vi "Dashboard Main.vi"() -> ()   [LabVIEW 2013]
uses:
  <vilib>/event_ctls.llb/eventvkey.ctl
  <vilib>/Rock Robotics/WPI/Dashboard/WPI_DashboardLogging Global.vi
  <vilib>/Utility/config.llb/Write Key (String).vi
  <vilib>/Utility/config.llb/Write Key (I32).vi
  <vilib>/Utility/config.llb/NI_LVConfig.lvlib
panel:
  out "Image Message":string="Timeout in Camera Communications"
  in  "Rec Mode":enum32{"Stop", "Record", "Playback"}(radio)
  in  "Dashboard Tab":T1(tab)
  in  "Camera Settings":T2={"Frame Rate"=30, "Compression"=30, "Size"=1} {"Frame Rate" scale=1.0..30.0; "Size" items=["640x480", "320x240", "160x120"]}
  out "MotorSliders R":cluster{"MotorSlide1":dbl, "MotorSlide2":dbl} {"MotorSlide2" scale=-1.0..1.0 scale format="%#_2e"; "MotorSlide1" scale=-1.0..1.0 scale format="%#_2e"}
  out "MotorChart R":cluster{"Numeric":dbl, "Numeric":dbl}(graph)
  out "MotorSliders L":T3 {"MotorSlide4 2" scale=0.0..14.0 scale format="%#_2e"; "MotorSlide2" scale=-1.0..1.0 scale format="%#_2e"; "MotorSlide1" scale=-1.0..1.0 scale format="%#_2e"}
  out "MotorChart L":T4(graph)
  out "JS1 Z":dbl(slide) scale=-1.0..1.0 scale format="%#_2e"
  out "Joystick 1":cluster{"X":dbl, "Y":dbl}[](graph)
  out "JS Buttons 1":T5
  out "JS2 Z":dbl(slide) scale=-1.0..1.0 scale format="%#_2e"
  out "Joystick 2":cluster{"X":dbl, "Y":dbl}[](graph)
  out "JS Buttons 2":T5
  out "Mode":T6(ring)=enum."Auto Disabled"
  out "Camera IP":string
  in  "DB Camera Config":bool
  out "fps":dbl format="%#.1g"
  out "Mbps":dbl format="%#.1g"
  out "Mbps 2":bool
  out "LED 1":bool
  in  "Light Ring On":bool
  in  "Drawback Pistons Activated":bool
  out "Buttons Of Same Pistons In Same State":bool
  in  "Compressor On/Off":bool
  in  "Grabber Pistons Extended":bool
  out "Are Grabber Pistons Extended":bool
  in  "Camera Pitch Control":dbl
  in  "Camera Rotation Control":dbl
  out "Is The Firing Pin Piston Extended":bool
  out "Are Drawback Pistons Extended":bool
  in  "Firing Pin Piston Extended":bool
  in  "Drawback Piston Extended":bool
  in  "Manual Mechanism Override":bool
  in  "Current Grabber Status":enum16{""}(ring)
  in  "Current Shooter Status":enum16{""}(ring)
  in  "Checkbox 2":bool
  in  "Checkbox 1":bool
  in  "Test Slider":dbl(slide) scale=0.0..100.0 scale format="%#_3g"
  in  "On/Off":bool caption="Solenoid"
  in  "Test Name":u16(ring) items=["Select the test to run...", "Example Test", "-------------------------------", "List of tests is built in robot code.", "Replace with your own automated tests."]
  in  "Test Tree":string(tree)
  in  "Motor":cluster{"Value":dbl, "Enable":bool} {"Value" scale=-1.0..1.0 scale format="%#_3g"}
  out "Progress":T7 {"Test Progress" scale=0.0..100.0}
  in  "Rev/Fwd":cluster{"Forward":bool, "Reverse":bool}
  in  "Test Ring":u16(ring) items=["Auto", "Fixed indoor", "Fixed outdoor 1", "Fixed outdoor 2", "Fixed fluorescent 1", "Fixed fluorescent 2", "Hold current"]
  in  "Listbox":i32(listbox)
  out "Tree":string(tree)
  out "Camera Image":T8(plugin-control)
  in  "Enable":bool
  # "Left"
  # "Front"
  # "Right"
  # "Battery"
  # "Don5"
  # "This tab is a great place for autonomous settings and validation.\nCustomize by placing controls and indicators here and name to\nmatch Dashboard Variables on robot."
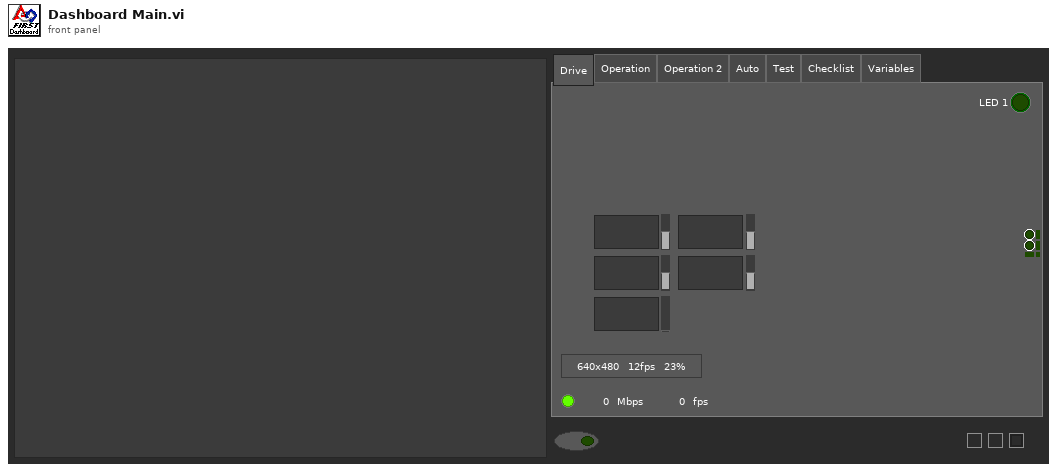
[diagram p1: front panel]
types:
  T1 = enum32{"Drive", "Operation", "Operation 2", "Auto", "Test", "Checklist", "Variables"}
  T2 = cluster{"Frame Rate":i32, "Compression":i32, "Size":u16}
  T3 = cluster{"MotorSlide1":dbl, "MotorSlide2":dbl, "MotorSlide4 2":dbl}
  T4 = cluster{"Numeric":dbl, "Numeric":dbl, "Battery":sgl}
  T5 = cluster{bool, bool, bool, bool, bool, bool, bool, bool, bool, bool, bool, bool}
  T6 = enum8{"Tele-Op Disabled", "Tele-Op Enabled", "Auto Disabled", "Auto Enabled", "Test Disabled", "Test Enabled", ""}
  T7 = cluster{"Test Progress":u8, "Test Progress Text":string}
  T8 = typedef "IMAQ Image.ctl" = refnum<image>
  T9 = enum32{"Drive", "Operation", "Auto", "Test", "Checklist", "Variables"}
  T10 = typedef "Image Type" = u32
  T11 = cluster{"Digital Inputs":bool[], "Digital Outputs":bool[]}
  T12 = cluster{"Competition mode":bool, "Robot Link":bool, "Autonomous":bool, "Enabled":bool, "E-Stop":bool, "Simulated":bool, "TestMode":bool, "Docked Window":bool}
  T13 = cluster{"Boolean Array[0]":bool, "Boolean Array[1]":bool, "Boolean Array[2]":bool, "Boolean Array[3]":bool, "Boolean Array[4]":bool, "Boolean Array[5]":bool, "Boolean Array[6]":bool, "Boolean Array[7]":bool, "Boolean Array[8]":bool, "Boolean Array[9]":bool, "Boolean Array[10]":bool, "Boolean Array[11]":bool}
  T14 = typedef "NI_LVConfig.lvlib/Config Data RefNum.ctl" = refnum<k1>
  T15 = typedef "eventvkey.ctl" = enum16{"ASCII", "Enter", "Return", "Shift", "Ctrl", "Alt", "Cmd", "Opt", "Caps", "NumLock", "Clear", "Break", "Up", "Down", "Left", "Right", "Insert", "Delete", "Home", "End", "PageUp", "PageDown", "Escape", "Help", "Pause", "ScrollLock", "F1", "F2", "F3", "F4", "F5", "F6", "F7", "F8", "F9", "F10", "F11", "F12", "F13", "F14", "F15", "F16", "F17", "F18", "F19", "F20", "F21", "F22", "F23", "F24", "Play", "VolumeUp", "VolumeDown", "Mute", "Two Byte Char"}
  T16 = cluster{"Image Size":bool, "Image Type":bool, "Pixel Value":bool, "ROI Information":bool, "Zoom Factor":bool}
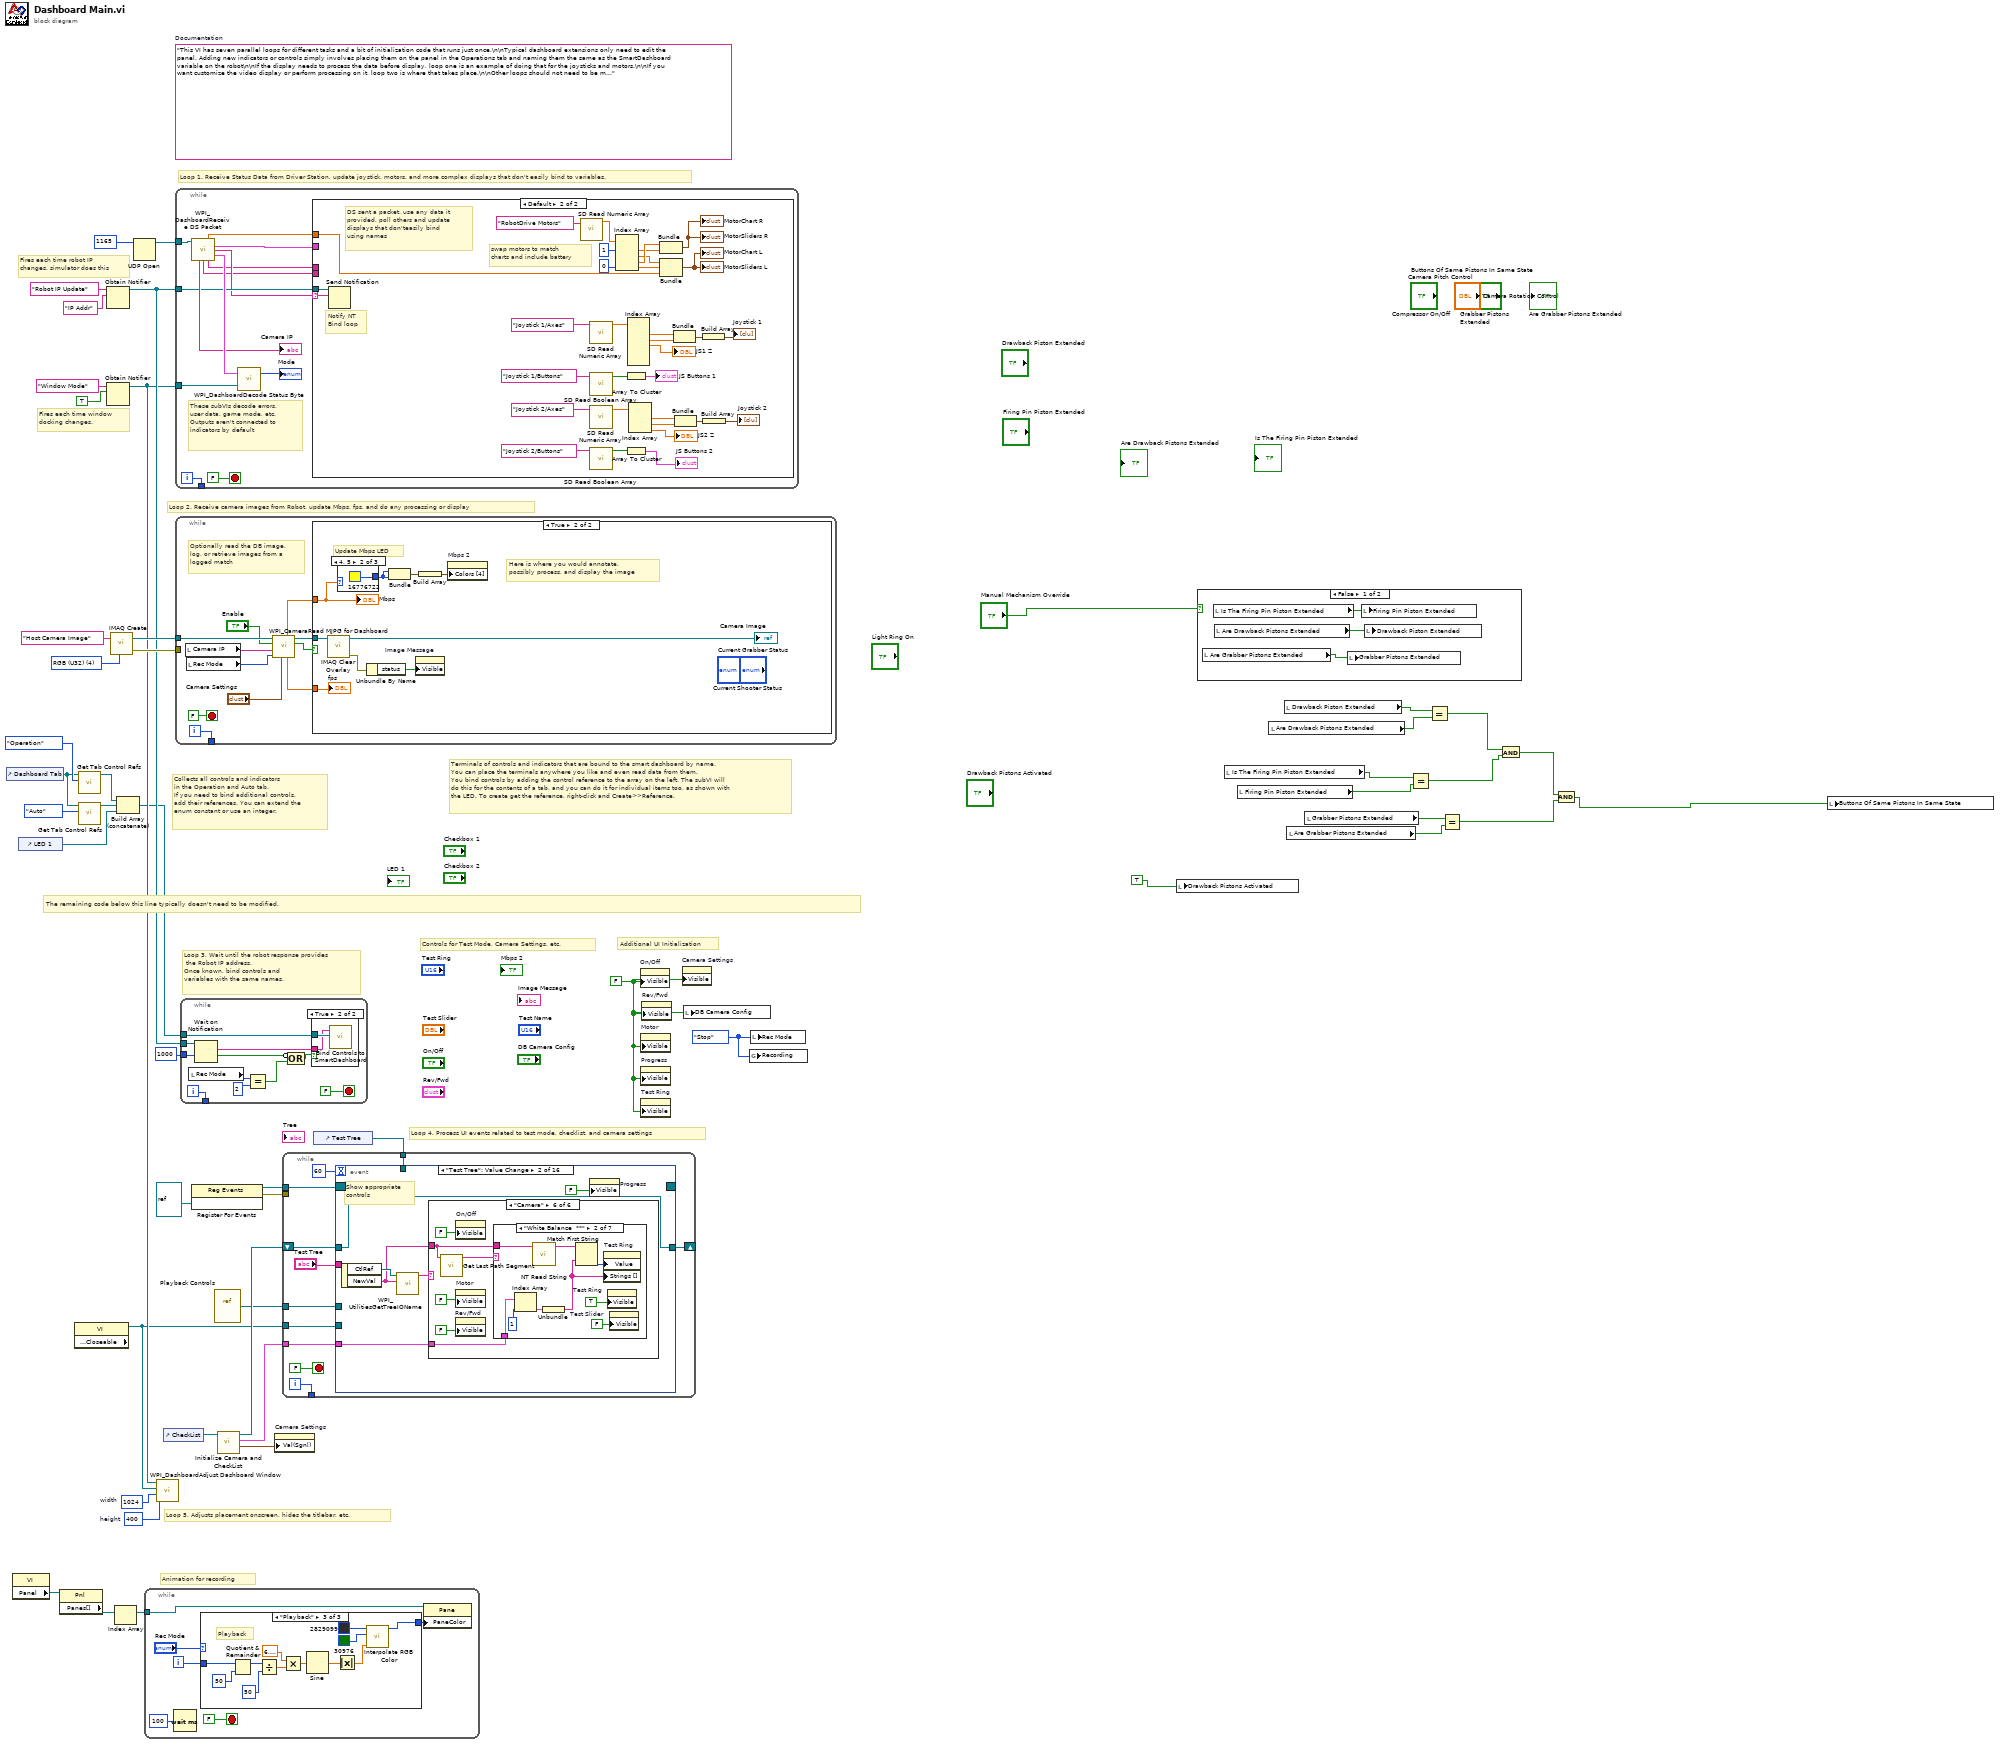
[diagram p0: block diagram]
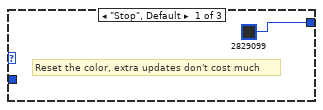
[diagram p3: hidden frame]
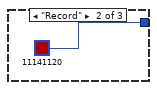
[diagram p4: hidden frame]
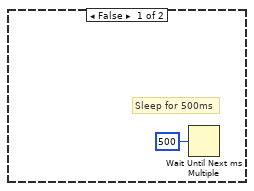
[diagram p6: hidden frame]
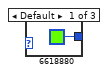
[diagram p7: hidden frame]
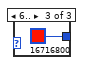
[diagram p8: hidden frame]
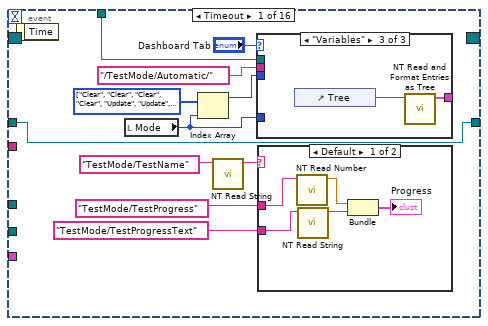
[diagram p9: hidden frame]
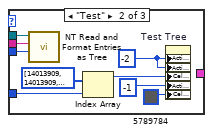
[diagram p11: hidden frame]
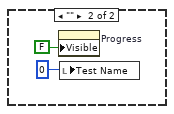
[diagram p12: hidden frame]
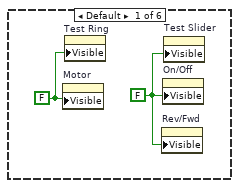
[diagram p13: hidden frame]
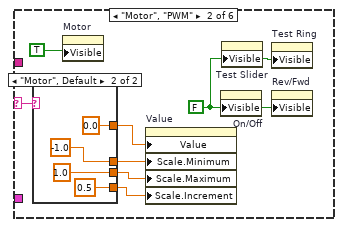
[diagram p14: hidden frame]
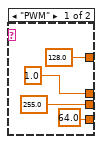
[diagram p15: hidden frame]
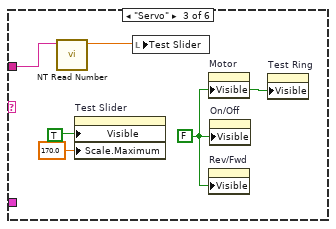
[diagram p16: hidden frame]
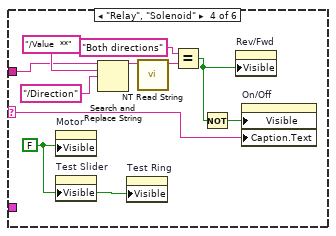
[diagram p17: hidden frame]
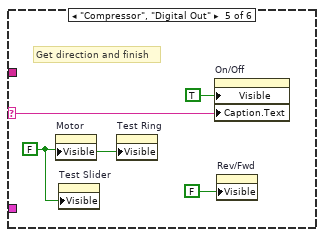
[diagram p18: hidden frame]
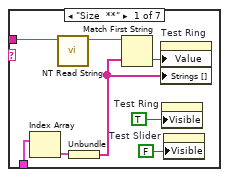
[diagram p19: hidden frame]
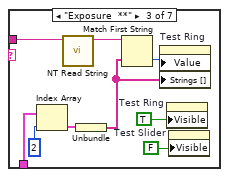
[diagram p20: hidden frame]
diagram:
  w21 = enum32{"Stop", "Record", "Playback"}."Stop" ("Rec Mode")
  w24 = 400  # height
  w25 = 1024  # width
  w38 = FALSE ("Visible")
  (unwired) "This VI has seven parallel loops for different tasks and a bit of initialization code that runs just once.\n\nTypical dashboard extensions only need to edit the panel. Adding new indicators or controls simply involves placing them on the panel in the Operations tab and naming them the same as the SmartDashboard variable on the robot\n\nIf the display needs to process the data before display, loop one is an example of doing that for the joysticks and motors.\n\nIf you want customize the video display or perform processing on it, loop two is where that takes place.\n\nOther loops should not need to be modified. They are pretty standard, and document the task they perform."  # Documentation
  w48 = T10 4 items=["Grayscale (U8)", "Grayscale (I16)", "Grayscale (SGL)", "Complex (CSG)", "RGB (U32)", "HSL (U32)", "RGB (U64)"] ("Image Type")
  # "Controls for Test Mode, Camera Settings, etc."
  # "Additional UI Initialization"
  # "Animation for recording"
  # "Fires each time robot IP\nchanges, simulator does this"
  # "Fires each time window\ndocking changes."
  # "Collects all controls and indicators\nin the Operation and Auto tab.\nIf you need to bind additional controls,\nadd their references. You can extend the\nenum constant or use an integer."
  # "The remaining code below this line typically doesn't need to be modified."
  # "Loop 4. Process UI events related to test mode, checklist, and camera settings"
  # "Terminals of controls and indicators that are bound to the smart dashboard by name.\nYou can place the terminals anywhere you like and even read data from them.\nYou bind controls by adding the control reference to the array on the left. The subVI will\ndo this for the contents of a tab, and you can do it for individual items too, as shown with\nthe LED. To create get the reference, right-click and Create>>Reference."
  # "Loop 3. Wait until the robot response provides\n the Robot IP address.\nOnce known, bind controls and\nvariables with the same names."
  # "Loop 5. Adjusts placement onscreen, hides the titlebar, etc."
  # "Loop 1. Receive Status Data from Driver Station, update joystick, motors, and more complex displays that don't easily bind to variables."
  # "Loop 2. Receive camera images from Robot, update Mbps, fps, and do any processing or display"
  n1 = control-ref of="Dashboard Tab"() -> (w19:refnum<vi>)
  n2 = property class="VI"() -> ("Panel"=w32:refnum<vi>)  [unwired: 2 in, 2 out]
  n3 = control-ref of="LED 1"() -> (w14:refnum<vi>)
  n4 = property class="Pnl"(reference=w32) -> ("Panes[]"=w33:refnum<vi>[])  [unwired: 1 in, 2 out]
  n5 = property class="VI" props=["Front Panel.Closeable"]() -> (reference out=w20:refnum<vi>)  [unwired: 2 in, 2 out]
  n6 = call <vilib>:"Get Tab Control Refs.vi"("Page Index"=T9."Operation" ("Dashboard Tab"), "TabControl in"=w19) -> ("ControlsOnPage"=w17:refnum<vi>[])  [unwired: 9 in]
  n7 = call <vilib>:"Get Tab Control Refs.vi"("Page Index"=T9."Auto" ("Dashboard Tab"), "TabControl in"=w19) -> ("ControlsOnPage"=w18:refnum<vi>[])  [unwired: 9 in]
  n8 = Obtain Notifier(name (unnamed)="Robot IP Update", notification data type="IP Addr" ("name (unnamed)")) -> (notifier out=w42:refnum<notifier>)  [unwired: 2 in, 2 out]
  n9 = Obtain Notifier(name (unnamed)="Window Mode", notification data type=TRUE) -> (notifier out=w23:refnum<notifier>)  [unwired: 2 in, 2 out]
  n10 = call "IMAQ Create"("Image Name"="Host Camera Image", "Image Type"=w48) -> ("New Image"=w46:T8, "error out"=w45:errorcluster)  [unwired: 2 in, 1 out]
  n11 = Index Array(array=w33) -> (element=w31:refnum<vi>)  [unwired: 1 in]
  n12 = Build Array (concatenate)(w17, w18, w14) -> (w16:refnum<vi>[])
  n13 = UDP Open(11:u16 1165 ("port")) -> (port=w49:refnum<k16>)  [unwired: 2 in, 4 out]
  n14 = while {
    tunnel: w31 -> [w52]
    i -> [w55]
    stop <- FALSE stop-if-true
    n15 = Wait (ms)(milliseconds to wait=u32 100) -> ()  [unwired: 1 out]
    n16 = case shown="\"Playback\"" "Rec Mode" {
      tunnel: w55 -> [_ _ w70]
      tunnel: [u32 2829099 ("Base Color") u32 11141120 ("Target Color") w59] -> w51
      frame "Stop", Default {
        # "Reset the color, extra updates don't cost much"
      }
      frame "Record" {
      }
      frame "Playback" {
        # "Playback"
        n17 = Quotient & Remainder(x=w70, y=u32 50 ("milliseconds to wait")) -> (x-y*floor(x/y)=w66:u32)  [unwired: 1 out]
        n18 = Divide(x=w66, y=u32 50 ("milliseconds to wait")) -> (x/y=w63:dbl)
        n19 = Multiply(x=6.283185307179586, y=w63) -> (x*y=w68:dbl)
        n20 = Sine(x=w68) -> (sin(x)=w67:dbl)
        n21 = Absolute Value(x=w67) -> (abs(x)=w60:dbl)
        n22 = call "Interpolate RGB Color.vi"("Proportion"=w60, "Target Color"=u32 30976, "Base Color"=u32 2829099) -> ("Result Color"=w59:u32)  [unwired: 8 in]
      }
    }
    n23 = property class="Pane"(reference=w52, "PaneColor"=w51) -> ()  [unwired: 1 in, 2 out]
  }
  n24 = call <vilib>:"WPI_DashboardAdjust Dashboard Window.vi"("height"=w24, "width"=w25, "reference in"=w20, "Notifier in"=w23) -> ()  [unwired: 8 in]
  n25 = control-ref of="CheckList"() -> (w22:refnum<vi>)
  n26 = while {
    tunnel: w46 -> [w79]
    tunnel: w45 -> [_]
    tunnel: [w80] -> _
    i -> [w80]
    stop <- FALSE stop-if-true
    # "Optionally read the DB image,\nlog, or retrieve images from a\nlogged match"
    n27 = local read "Camera IP"() -> (w72:string)
    n28 = local read "Rec Mode"() -> (w71:enum32{"Stop", "Record", "Playback"})
    n29 = call <vilib>:"WPI_CameraRead MJPG for Dashboard.vi"("Camera Settings"="Camera Settings", "Rec Mode"=w71, "Camera IP"=w72, "Enable"="Enable", "Refnum in"=w79) -> ("Active"=w76:bool, "Refnum out"=w78:T8, "FPS"=w75:dbl, "Bandwidth (Mbps)"=w74:dbl)  [unwired: 3 in]
    n30 = case shown="True" w76 {
      tunnel: w78 -> [_ w86]
      tunnel: w74 -> [_ w85]
      tunnel: w75 -> [_ w83]
      frame False {
        # "Sleep for 500ms"
        n31 = Wait Until Next ms Multiple(millisecond multiple=u32 500) -> ()  [unwired: 1 out]
      }
      frame True {
        # "Here is where you would annotate,\npossibly process, and display the image"
        # "Update Mbps LED"
        n32 = call "IMAQ Clear Overlay"("Image"=w86) -> ("error out"=w90:errorcluster, "Image Out"=→"Camera Image":T8)  [unwired: 2 in, 7 out]
        n33 = case shown="4, 5" w85 {
          tunnel: [u32 6618880 ("Color Box") u32 16776722 ("Color Box") u32 16716800 ("Color Box")] -> w87
          frame Default {
          }
          frame 4, 5 {
          }
          frame 6.. {
          }
        }
        n34 = Unbundle By Name(w90) -> ("status"=w91:bool)
        n35 = Bundle("Color Box"=w87, "Color Box"=w87) -> (w89:cluster{"Color Box":u32, "Color Box":u32})  [unwired: 1 out]
        n36 = property on="Image Message" class="Str"("Visible"=w91) -> ()  [unwired: 2 in, 2 out]
        n37 = Build Array(w89) -> (w88:cluster{"Color Box":u32, "Color Box":u32}[])
        n38 = property on="Mbps 2" class="Bool (strict)"("Colors [4]"=w88) -> ()  [unwired: 2 in, 2 out]
        "Mbps" <- w85
        "fps" <- w83
      }
    }
  }
  n39 = while {
    tunnel: w49 -> [w105]
    tunnel: w42 -> [w100]
    tunnel: w23 -> [w104]
    tunnel: [w101] -> _
    i -> [w101]
    stop <- FALSE stop-if-true
    # "These subVIs decode errors, user data, game mode, etc.\nOutputs aren't connected to indicators by default"
    n40 = call <vilib>:"WPI_DashboardReceive DS Packet.vi"("Recv Socket"=w105) -> ("Battery"=w95:sgl, "Driver Station"=w96:T11, "Robot IP Address"=w99:string, "Status"=w106:T12, "Camera IP Address"=→"Camera IP":string, "Low Priority User Data"=w98:string, "High Priority User Data"=w97:string)  [unwired: 1 in, 7 out]
    n41 = call <vilib>:"WPI_DashboardDecode Status Byte.vi"("Window Mode Notifier"=w104, "Status"=w106) -> ("Mode"=→"Mode":T6)  [unwired: 1 out]
    n42 = case shown="Default" w99 {
      selector: w99 -> [_ w118]
      tunnel: w100 -> [_ w119]
      tunnel: w98 -> [_ _]
      tunnel: w97 -> [_ _]
      tunnel: w96 -> [_ _]
      tunnel: w95 -> [_ w117]
      frame "0.0.0.0" {
        # "DS not sending packets, or no robot exists yet.\nDon't poll the variables"
      }
      frame Default {
        # "Notify NT\nBind loop"
        # "DS sent a packet. use any data it\nprovided, poll others and update\ndisplays that don'teasily bind\nusing names"
        # "swap motors to match\ncharts and include battery"
        n43 = Send Notification(notification=w118, notifier=w119) -> ()  [unwired: 1 in, 2 out]
        n44 = call <vilib>:"SD Read Numeric Array.vi"("Name"="RobotDrive Motors") -> ("Numeric Array"=w116:dbl[])  [unwired: 8 in, 2 out]
        n45 = call <vilib>:"SD Read Numeric Array.vi"("Name"="Joystick 1/Axes") -> ("Numeric Array"=w135:dbl[])  [unwired: 8 in, 2 out]
        n46 = call <vilib>:"SD Read Boolean Array.vi"("Name"="Joystick 1/Buttons") -> ("Boolean Array"=w137:bool[])  [unwired: 8 in, 2 out]
        n47 = call <vilib>:"SD Read Numeric Array.vi"("Name"="Joystick 2/Axes") -> ("Numeric Array"=w129:dbl[])  [unwired: 8 in, 2 out]
        n48 = call <vilib>:"SD Read Boolean Array.vi"("Name"="Joystick 2/Buttons") -> ("Boolean Array"=w128:bool[])  [unwired: 8 in, 2 out]
        n49 = Index Array(array=w116, index #1=1, index #4=0) -> (element #1=w112:dbl, element #2=w111:dbl, element #3=w113:dbl, element #4=w108:dbl)  [unwired: 2 in]
        n50 = Array To Cluster(array=w137) -> (cluster=→"JS Buttons 1":T13)
        n51 = Array To Cluster(array=w128) -> (cluster=→"JS Buttons 2":T13)
        n52 = Index Array(array=w135) -> (element #1=w132:dbl, element #2=w133:dbl, element #3=→"JS1 Z":dbl)  [unwired: 6 in, 3 out]
        n53 = Index Array(array=w129) -> (element #1=w124:dbl, element #2=w123:dbl, element #3=→"JS2 Z":dbl)  [unwired: 3 in]
        n54 = Bundle("Numeric"=w113, "Numeric"=w112) -> (→"MotorChart R" →"MotorSliders R":cluster{"Numeric":dbl, "Numeric":dbl})  [unwired: 1 in]
        n55 = Bundle("Numeric"=w111, "Numeric"=w108, "Battery"=w117) -> (→"MotorChart L" →"MotorSliders L":T4)  [unwired: 1 in]
        n56 = Bundle("Numeric"=w132, "Numeric"=w133) -> (w131:cluster{"Numeric":dbl, "Numeric":dbl})  [unwired: 1 in]
        n57 = Bundle("Numeric"=w124, "Numeric"=w123) -> (w125:cluster{"Numeric":dbl, "Numeric":dbl})  [unwired: 1 in]
        n58 = Build Array(w131) -> (→"Joystick 1":cluster{"Numeric":dbl, "Numeric":dbl}[])
        n59 = Build Array(w125) -> (→"Joystick 2":cluster{"Numeric":dbl, "Numeric":dbl}[])
      }
    }
  }
  n60 = while {
    tunnel: w16 -> [w151]
    tunnel: w42 -> [w149]
    tunnel: [w147] -> _
    tunnel: u32 1000 ("milliseconds to wait") -> [w146]
    i -> [w147]
    stop <- FALSE stop-if-true
    n61 = local read "Rec Mode"() -> (w142:enum32{"Stop", "Record", "Playback"})
    n62 = Wait on Notification(notifier=w149, timeout in ms (-1)=w146) -> (notification=w148:string, timed out?=w144:bool)  [unwired: 2 in, 2 out]
    n63 = Equal?(x=w142, y=u16 2 ("Rec Mode")) -> (x = y?=w143:bool)
    n64 = Compound Arithmetic op=OR(invert w144, w143) -> (w145:bool)
    n65 = case shown="True" w145 {
      tunnel: w151 -> [_ w153]
      tunnel: w148 -> [_ w152]
      frame False {
      }
      frame True {
        n66 = call <vilib>:"Bind Controls to SmartDashboard.vi"("Bound Control Refs"=w153, "Server IP Address"=w152) -> ()  [unwired: 10 in]
      }
    }
  }
  n67 = register-events(refnum<vi> refnum) -> (reference out=w29:refnum<event-registration>, error out=w28:errorcluster)  [unwired: 2 in]
  n68 = vi-ref "Playback Controls.vi"() -> (w30:refnum<vi>)
  n69 = call "Initialize Camera and CheckList.vi"("ListBox in"=w22) -> ("Cluster"=w36:cluster{"value":i32, "value":i32, "index":i32}, "Array"=w37:cluster{string[]}[], "File Refnum"=w35:T14)  [unwired: 8 in]
  n70 = property on="Camera Settings" class="Clust (strict)"("Val(Sgnl)"=w36) -> ()  [unwired: 2 in, 2 out]
  n71 = control-ref of="Test Tree"() -> (w34:refnum<vi>)
  n72 = while {
    tunnel: w37 -> [w161]
    shift-right: [w160] -> _
    shift-left: w35 -> [w159]
    tunnel: [w158] -> _
    tunnel: w34 -> [w157]
    tunnel: w30 -> [w156]
    tunnel: w29 -> [w155]
    tunnel: w28 -> [_]
    tunnel: w20 -> [w154]
    i -> [w158]
    stop <- FALSE stop-if-true
    n73 = event shown="[1] \"Test Tree\": Value Change" {
      selector: w155 -> [_ _ _ _ _ _ _ _ _ _ _ _ _ _ _ _]
      dyn-events: [_ _ _ _ _ _ _ _ _ _ _ _ _ w399 _ _] -> _
      timeout: u32 60 ("milliseconds to wait") -> [_ _ _ _ _ _ _ _ _ _ _ _ _ _ _ _]
      tunnel: w157 -> [w171 _ _ _ _ _ _ _ _ _ _ _ _ _ _ _]
      tunnel: "Test Tree" -> [_ _ _ _ _ _ _ _ w368 w376 w378 w382 w390 _ _ _]
      tunnel: w161 -> [_ w195 _ _ _ _ w332 w362 _ _ _ _ _ _ _ _]
      tunnel: [w165 w194 w293 w298 w306 w318 w331 w355 w367 w374 w377 w381 w389 w401 w415 w416] -> w160
      tunnel: w159 -> [w165 w194 w293 w298 w306 w318 w330 w355 w367 w374 w377 w381 w389 w401 w415 w416]
      tunnel: w156 -> [_ _ _ _ _ _ _ _ _ _ _ _ _ w402 _ w419]
      tunnel: w154 -> [_ _ _ _ _ _ _ _ _ _ _ _ _ w397 _ _]
      event Timeout {
        w170 = enum16{"Update", "Clear"}[] [enum."Clear", enum."Clear", enum."Clear", enum."Clear", enum."Update", enum."Update", enum."Clear"] items=["Update", "Clear"]
        n74 = event-data() -> ()  [unwired: 1 in, 1 out]
        n75 = local read "Mode"() -> (w168:T6)
        n76 = Index Array(array=w170, index=w168) -> (element=w169:enum16{"Update", "Clear"})
        n77 = call <vilib>:"NT Read String.vi"("Name"="TestMode/TestName") -> ("String"=w174:string)  [unwired: 9 in, 1 out]
        n78 = case shown="\"Variables\"" "Dashboard Tab" {
          tunnel: w171 -> [_ w184 _]
          tunnel: "/TestMode/Automatic/" ("Name Pattern") -> [_ w183 _]
          tunnel: w169 -> [_ w182 _]
          tunnel: w168 -> [_ w180 _]
          tunnel: [_ _ w186] -> _
          frame "Operation", Default {
          }
          frame "Test" {
            w179 = -2 ("Active Item:Row Number")
            n79 = call <vilib>:"NT Read and Format Entries as Tree.vi"("Operation"=w182, "Name Pattern"=w183, "Tree Refnum"=w184) -> ()  [unwired: 7 in, 2 out]
            n80 = Index Array(array=u32[] [14013909, 14013909, 14013909, 14013909, 14013909, 16777215, 14013909], index=w180) -> (element=w178:u32)
            n81 = property on="Test Tree" class="Tree (strict)"("Active Item Row Number"=w179, "ActiveColNum"=w179, "CellBG"=w178, "Active Item Row Number"=-1 ("Active Item:Row Number"), "CellBG"=u32 5789784 ("Color Box")) -> ()  [unwired: 2 in, 2 out]
          }
          frame "Variables" {
            n82 = control-ref of="Tree"() -> (w185:refnum<vi>)
            n83 = call <vilib>:"NT Read and Format Entries as Tree.vi"("Tree Refnum"=w185) -> ("Formatted Strings"=w186:cluster{"Name":string, "Value":string}[])  [unwired: 9 in, 1 out]
          }
        }
        n84 = case shown="Default" w174 {
          tunnel: "TestMode/TestProgress" ("Name") -> [w188 _]
          tunnel: "TestMode/TestProgressText" ("Name") -> [w187 _]
          frame Default {
            n85 = call <vilib>:"NT Read Number.vi"("Name"=w188) -> ("Numeric"=w189:dbl)  [unwired: 9 in, 1 out]
            n86 = call <vilib>:"NT Read String.vi"("Name"=w187) -> ("String"=w190:string)  [unwired: 9 in, 1 out]
            n87 = Bundle("Numeric"=w189, "String"=w190) -> (→"Progress":cluster{"Numeric":dbl, "String":string})  [unwired: 1 in]
          }
          frame "" {
            n88 = property on="Progress" class="Clust (strict)"("Visible"=FALSE) -> ()  [unwired: 2 in, 2 out]
            n89 = local write "Test Name"(u16 0) -> ()
          }
        }
      }
      event "Test Tree": Value Change {
        # "Show appropriate\ncontrols"
        n90 = event-data() -> ("CtlRef"=w198:refnum<vi>, "NewVal"=w196:string)  [unwired: 1 in]
        n91 = call <vilib>:"WPI_UtilitiesGetTreeIOName.vi"("NewVal"=w196, "TreeControl in"=w198) -> ("I/O Name"=w199:string)  [unwired: 9 in]
        n92 = case shown="\"Camera\"" w199 {
          selector: w199 -> [_ w206 _ w224 w233 _]
          tunnel: w196 -> [_ _ w221 w223 _ w240]
          tunnel: w195 -> [_ _ _ _ _ w239]
          frame Default {
            w201 = FALSE ("Visible")
            w200 = FALSE ("Visible")
            n93 = property on="Motor" class="Clust (strict)"("Visible"=w200) -> ()  [unwired: 2 in, 2 out]
            n94 = property on="Test Ring" class="Ring (strict)"("Visible"=w200) -> ()  [unwired: 2 in, 2 out]
            n95 = property on="Rev/Fwd" class="Clust (strict)"("Visible"=w201) -> ()  [unwired: 2 in, 2 out]
            n96 = property on="On/Off" class="Bool (strict)"("Visible"=w201) -> ()  [unwired: 2 in, 2 out]
            n97 = property on="Test Slider" class="Slide (strict)"("Visible"=w201) -> ()  [unwired: 2 in, 2 out]
          }
          frame "Motor", "PWM" {
            w207 = FALSE ("Visible")
            n98 = case shown="\"Motor\", Default" w206 {
              tunnel: [1.0 ("Value") -1.0 ("Value")] -> w205
              tunnel: [255.0 ("Value") 1.0 ("Value")] -> w204
              tunnel: [128.0 ("Value") 0.0 ("Value")] -> w203
              tunnel: [64.0 ("Value") 0.5 ("Value")] -> w202
              frame "PWM" {
              }
              frame "Motor", Default {
              }
            }
            n99 = property on="Motor" class="Clust (strict)"("Visible"=TRUE) -> ()  [unwired: 2 in, 2 out]
            n100 = property on="Value" class="Slide (strict)"("Value"=w203, "Scale.Minimum"=w205, "Scale.Maximum"=w204, "Scale.Increment"=w202) -> ()  [unwired: 2 in, 2 out]
            n101 = property on="On/Off" class="Bool (strict)"("Visible"=w207) -> ()  [unwired: 2 in, 2 out]
            n102 = property on="Test Slider" class="Slide (strict)"("Visible"=w207) -> ()  [unwired: 2 in, 2 out]
            n103 = property on="Test Ring" class="Ring (strict)"("Visible"=w207) -> ()  [unwired: 2 in, 2 out]
            n104 = property on="Rev/Fwd" class="Clust (strict)"("Visible"=w207) -> ()  [unwired: 2 in, 2 out]
          }
          frame "Servo" {
            w219 = FALSE ("Visible")
            n105 = call <vilib>:"NT Read Number.vi"("Name"=w221) -> ("Numeric"=w220:dbl)  [unwired: 9 in, 1 out]
            n106 = property on="Test Slider" class="Slide (strict)"("Visible"=TRUE, "Scale.Maximum"=170.0 ("Scale.Range:Maximum")) -> ()  [unwired: 2 in, 2 out]
            n107 = local write "Test Slider"(w220) -> ()
            n108 = property on="Motor" class="Clust (strict)"("Visible"=w219) -> ()  [unwired: 2 in, 2 out]
            n109 = property on="Rev/Fwd" class="Clust (strict)"("Visible"=w219) -> ()  [unwired: 2 in, 2 out]
            n110 = property on="On/Off" class="Bool (strict)"("Visible"=w219) -> ()  [unwired: 2 in, 2 out]
            n111 = property on="Test Ring" class="Ring (strict)"("Visible"=w219) -> ()  [unwired: 2 in, 2 out]
          }
          frame "Relay", "Solenoid" {
            w222 = FALSE ("Visible")
            n112 = property on="Motor" class="Clust (strict)"("Visible"=w222) -> ()  [unwired: 2 in, 2 out]
            n113 = property on="Test Slider" class="Slide (strict)"("Visible"=w222) -> ()  [unwired: 2 in, 2 out]
            n114 = Search and Replace String(input string=w223, search string="/Value  **", replace string="/Direction") -> (result string=w229:string)  [unwired: 5 in, 3 out]
            n115 = property on="Test Ring" class="Ring (strict)"("Visible"=w222) -> ()  [unwired: 2 in, 2 out]
            n116 = call <vilib>:"NT Read String.vi"("Name"=w229) -> ("String"=w227:string)  [unwired: 9 in, 1 out]
            n117 = Equal?(x="Both directions", y=w227) -> (x = y?=w225:bool)
            n118 = Not(x=w225) -> (.not. x?=w226:bool)
            n119 = property on="Rev/Fwd" class="Clust (strict)"("Visible"=w225) -> ()  [unwired: 2 in, 2 out]
            n120 = property on="On/Off" class="Bool (strict)"("Visible"=w226, "Caption.Text"=w224) -> ()  [unwired: 2 in, 2 out]
          }
          frame "Compressor", "Digital Out" {
            w232 = FALSE ("Visible")
            # "Get direction and finish"
            n121 = property on="Motor" class="Clust (strict)"("Visible"=w232) -> ()  [unwired: 2 in, 2 out]
            n122 = property on="Test Slider" class="Slide (strict)"("Visible"=w232) -> ()  [unwired: 2 in, 2 out]
            n123 = property on="Test Ring" class="Ring (strict)"("Visible"=w232) -> ()  [unwired: 2 in, 2 out]
            n124 = property on="On/Off" class="Bool (strict)"("Visible"=TRUE, "Caption.Text"=w233) -> ()  [unwired: 2 in, 2 out]
            n125 = property on="Rev/Fwd" class="Clust (strict)"("Visible"=FALSE) -> ()  [unwired: 2 in, 2 out]
          }
          frame "Camera" {
            n126 = call <vilib>:"Get Last Path Segment.vi"("String in"=w240) -> ("String out"=w241:string)  [unwired: 10 in]
            n127 = property on="On/Off" class="Bool (strict)"("Visible"=FALSE) -> ()  [unwired: 2 in, 2 out]
            n128 = property on="Motor" class="Clust (strict)"("Visible"=FALSE) -> ()  [unwired: 2 in, 2 out]
            n129 = property on="Rev/Fwd" class="Clust (strict)"("Visible"=FALSE) -> ()  [unwired: 2 in, 2 out]
            n130 = case shown="\"White Balance  **\"" w241 {
              tunnel: w240 -> [w247 w256 w265 w274 w283 _ w289]
              tunnel: w239 -> [w245 w253 w262 w271 w280 _ _]
              frame "Size  **" {
                n131 = Index Array(array=w245) -> (element=w244:cluster{string[]})  [unwired: 1 in]
                n132 = call <vilib>:"NT Read String.vi"("Name"=w247) -> ("String"=w246:string)  [unwired: 9 in, 1 out]
                n133 = Unbundle(w244) -> (w242:string[])
                n134 = Match First String(2:w242, 3:w246) -> (0:w243:i32)  [unwired: 1 out]
                n135 = property on="Test Ring" class="Ring (strict)"("Value"=w243, "Strings []"=w242) -> ()  [unwired: 2 in, 2 out]
                n136 = property on="Test Ring" class="Ring (strict)"("Visible"=TRUE) -> ()  [unwired: 2 in, 2 out]
                n137 = property on="Test Slider" class="Slide (strict)"("Visible"=FALSE) -> ()  [unwired: 2 in, 2 out]
              }
              frame "White Balance  **" {
                n138 = Index Array(array=w253, index=1) -> (element=w254:cluster{string[]})
                n139 = call <vilib>:"NT Read String.vi"("Name"=w256) -> ("String"=w255:string)  [unwired: 9 in, 1 out]
                n140 = Unbundle(w254) -> (w251:string[])
                n141 = Match First String(2:w251, 3:w255) -> (0:w250:i32)  [unwired: 1 out]
                n142 = property on="Test Ring" class="Ring (strict)"("Value"=w250, "Strings []"=w251) -> ()  [unwired: 2 in, 2 out]
                n143 = property on="Test Ring" class="Ring (strict)"("Visible"=TRUE) -> ()  [unwired: 2 in, 2 out]
                n144 = property on="Test Slider" class="Slide (strict)"("Visible"=FALSE) -> ()  [unwired: 2 in, 2 out]
              }
              frame "Exposure  **" {
                n145 = Index Array(array=w262, index=2) -> (element=w263:cluster{string[]})
                n146 = call <vilib>:"NT Read String.vi"("Name"=w265) -> ("String"=w264:string)  [unwired: 9 in, 1 out]
                n147 = Unbundle(w263) -> (w259:string[])
                n148 = Match First String(2:w259, 3:w264) -> (0:w260:i32)  [unwired: 1 out]
                n149 = property on="Test Ring" class="Ring (strict)"("Value"=w260, "Strings []"=w259) -> ()  [unwired: 2 in, 2 out]
                n150 = property on="Test Ring" class="Ring (strict)"("Visible"=TRUE) -> ()  [unwired: 2 in, 2 out]
                n151 = property on="Test Slider" class="Slide (strict)"("Visible"=FALSE) -> ()  [unwired: 2 in, 2 out]
              }
              frame "Exposure Priority  **" {
                n152 = Index Array(array=w271, index=3) -> (element=w272:cluster{string[]})
                n153 = call <vilib>:"NT Read String.vi"("Name"=w274) -> ("String"=w273:string)  [unwired: 9 in, 1 out]
                n154 = Unbundle(w272) -> (w268:string[])
                n155 = Match First String(2:w268, 3:w273) -> (0:w269:i32)  [unwired: 1 out]
                n156 = property on="Test Ring" class="Ring (strict)"("Value"=w269, "Strings []"=w268) -> ()  [unwired: 2 in, 2 out]
                n157 = property on="Test Ring" class="Ring (strict)"("Visible"=TRUE) -> ()  [unwired: 2 in, 2 out]
                n158 = property on="Test Slider" class="Slide (strict)"("Visible"=FALSE) -> ()  [unwired: 2 in, 2 out]
              }
              frame "Color Enable  **" {
                n159 = Index Array(array=w280, index=4) -> (element=w281:cluster{string[]})
                n160 = call <vilib>:"NT Read String.vi"("Name"=w283) -> ("String"=w282:string)  [unwired: 9 in, 1 out]
                n161 = Unbundle(w281) -> (w277:string[])
                n162 = Match First String(2:w277, 3:w282) -> (0:w278:i32)  [unwired: 1 out]
                n163 = property on="Test Ring" class="Ring (strict)"("Value"=w278, "Strings []"=w277) -> ()  [unwired: 2 in, 2 out]
                n164 = property on="Test Ring" class="Ring (strict)"("Visible"=TRUE) -> ()  [unwired: 2 in, 2 out]
                n165 = property on="Test Slider" class="Slide (strict)"("Visible"=FALSE) -> ()  [unwired: 2 in, 2 out]
              }
              frame Default {
                n166 = property on="Test Ring" class="Ring (strict)"("Visible"=FALSE) -> ()  [unwired: 2 in, 2 out]
                n167 = property on="Test Slider" class="Slide (strict)"("Visible"=FALSE) -> ()  [unwired: 2 in, 2 out]
              }
              frame "Brightness  **", "Color Level  **", "Compression  **", "FPS  **", "Sharpness  **" {
                n168 = call <vilib>:"NT Read Number.vi"("Name"=w289) -> ("Numeric"=w288:dbl)  [unwired: 9 in, 1 out]
                n169 = local write "Test Slider"(w288) -> ()
                n170 = property on="Test Slider" class="Slide (strict)"("Visible"=TRUE, "Scale.Maximum"=100.0 ("Scale.Range:Maximum")) -> ()  [unwired: 2 in, 2 out]
                n171 = property on="Test Ring" class="Ring (strict)"("Visible"=FALSE) -> ()  [unwired: 2 in, 2 out]
              }
            }
          }
        }
        n172 = property on="Progress" class="Clust (strict)"("Visible"=FALSE) -> ()  [unwired: 2 in, 2 out]
      }
      event "Test Name": Mouse Enter {
        # "Populate the ring with the list of tests"
        n173 = event-data() -> ()  [unwired: 1 in, 1 out]
        n174 = call <vilib>:"NT Read String Array.vi"("Name"="TestMode/TestList") -> ("String Array"=w297:string[])  [unwired: 9 in, 1 out]
        n175 = Build Array (concatenate)("Select the test to run...", w297) -> (w296:string[])
        n176 = property on="Test Name" class="Ring (strict)"("Strings []"=w296) -> ()  [unwired: 2 in, 2 out]
      }
      event "Test Name": Value Change {
        w299 = FALSE ("Visible")
        # "Tell the robot the test name to run"
        n177 = event-data() -> ("NewVal"=w303:u16)  [unwired: 1 in]
        n178 = property on="Test Name" class="Ring (strict)"() -> ("Strings []"=w304:string[])  [unwired: 2 in, 2 out]
        n179 = local write "Progress"(T7 {"Test Progress"=0, "Test Progress Text"=""} ("Progress")) -> ()
        n180 = Index Array(array=w304, index=w303) -> (element=w302:string)
        n181 = call <vilib>:"NT Write String.vi"("String"=w302, "Name"="TestMode/TestName") -> ()  [unwired: 9 in, 1 out]
        n182 = property on="Progress" class="Clust (strict)"("Visible"=TRUE) -> ()  [unwired: 2 in, 2 out]
        n183 = property on="Motor" class="Clust (strict)"("Visible"=w299) -> ()  [unwired: 2 in, 2 out]
        n184 = property on="Test Slider" class="Slide (strict)"("Visible"=w299) -> ()  [unwired: 2 in, 2 out]
        n185 = property on="On/Off" class="Bool (strict)"("Visible"=w299) -> ()  [unwired: 2 in, 2 out]
        n186 = property on="Rev/Fwd" class="Clust (strict)"("Visible"=w299) -> ()  [unwired: 2 in, 2 out]
        n187 = property on="Test Ring" class="Ring (strict)"("Visible"=w299) -> ()  [unwired: 2 in, 2 out]
      }
      event "Listbox": Double Click {
        n188 = event-data() -> ("PlatMods.Shift"=w307:bool, "Row"=w309:i32)  [unwired: 1 in]
        n189 = case shown="True" w307 {
          tunnel: w309 -> [w313 _]
          tunnel: 1 -> [w312 _]
          frame False {
            n190 = property on="Listbox" class="LstBox (strict)"() -> ("Item Symbols"=w311:i32[])  [unwired: 2 in, 2 out]
            n191 = Replace Array Subset(array=w311, new element=w312, index=w313) -> (w310:i32[])
            n192 = property on="Listbox" class="LstBox (strict)"("Item Symbols"=w310) -> ()  [unwired: 2 in, 2 out]
          }
          frame True {
            w314 = 0 ("Top Row")
            n193 = property on="Listbox" class="LstBox (strict)"() -> ("Number of Rows"=w316:u32)  [unwired: 2 in, 2 out]
            n194 = Initialize Array(0, w316) -> (w315:i32[])
            n195 = property on="Listbox" class="LstBox (strict)"("Top Row"=w314, "Value"=w314, "Item Symbols"=w315) -> ()  [unwired: 2 in, 2 out]
          }
        }
      }
      event "Listbox": Key Down {
        n196 = event-data() -> ("VKey"=w320:T15)  [unwired: 1 in]
        n197 = case shown="\"Left\", \"Right\"" w320 {
          selector: w320 -> [w325 _]
          tunnel: eventvkey."Left" ("VKey") -> [w323 _]
          frame "Left", "Right" {
            n198 = Equal?(x=w323, y=w325) -> (x = y?=w324:bool)
            n199 = Select(t=0, s=w324, f=1) -> (s? t:f=w326:i32)
            n200 = property on="Listbox" class="LstBox (strict)"() -> ("Item Symbols"=w329:i32[])  [unwired: 2 in, 2 out]
            n201 = Replace Array Subset(array=w329, new element=w326, index="Listbox") -> (w328:i32[])
            n202 = property on="Listbox" class="LstBox (strict)"("Item Symbols"=w328) -> ()  [unwired: 2 in, 2 out]
          }
          frame Default {
          }
        }
      }
      event "DB Camera Config": Value Change {
        n203 = event-data() -> ("NewVal"=w333:bool)  [unwired: 1 in]
        n204 = case shown="False" w333 {
          tunnel: w332 -> [w342 _]
          tunnel: [w335 w353] -> w331
          tunnel: w330 -> [w334 w353]
          frame False {
            w349 = "Camera"
            w352 = FALSE ("Visible")
            n205 = local read "Camera Settings"() -> (w341:T2)
            n206 = Index Array(array=w342) -> (element=w345:cluster{string[]})  [unwired: 1 in]
            n207 = Unbundle(w341) -> ("Frame Rate"=w340:i32, "Compression"=w339:i32, "Size"=w343:u16)
            n208 = Unbundle(w345) -> (w344:string[])
            n209 = Index Array(array=w344, index=w343) -> (element=w338:string)
            n210 = call-poly <vilib>:"Write Key.vi"("section"=w349, "value"=w338, "key"="Size", "refnum"=w334) -> ("refnum out"=w351:T14)  [unwired: 2 in, 5 out]
            n211 = call-poly <vilib>:"Write Key.vi"("section"=w349, "value"=w340, "key"="FrameRate", "refnum"=w351) -> ("refnum out"=w350:T14)  [unwired: 1 in, 6 out]
            n212 = property on="Camera Settings" class="Clust (strict)"("Visible"=w352) -> ()  [unwired: 2 in, 2 out]
            n213 = local write "DB Camera Config"(w352) -> ()
            n214 = call-poly <vilib>:"Write Key.vi"("section"=w349, "value"=w339, "key"="Compression", "refnum"=w350) -> ("refnum out"=w336:T14)  [unwired: 1 in, 6 out]
            n215 = call <vilib>:"Close Config Data.vi"("refnum"=w336) -> ("file path"=w337:path)  [unwired: 2 in, 8 out]
            n216 = call <vilib>:"Open Config Data.vi"("configuration file path"=w337) -> ("refnum"=w335:T14)  [unwired: 8 in, 2 out]
          }
          frame True {
            n217 = property on="Camera Settings" class="Clust (strict)"("Visible"=TRUE) -> ()  [unwired: 2 in, 2 out]
          }
        }
      }
      event "Camera Settings": Value Change {
        n218 = event-data() -> ("NewVal"=w366:T2)  [unwired: 1 in]
        n219 = Index Array(array=w362) -> (element=w361:cluster{string[]})  [unwired: 1 in]
        n220 = Unbundle(w366) -> ("Frame Rate"=w357:i32, "Compression"=w356:i32, "Size"=w359:u16)
        n221 = Unbundle(w361) -> (w360:string[])
        n222 = Index Array(array=w360, index=w359) -> (element=w358:string)
        n223 = Format Into String(format string="%s   %dfps   %d%%", w358, w357, w356) -> (resulting string=w363:string)  [unwired: 2 in, 1 out]
        n224 = Build Array(w363) -> (w364:string[])
        n225 = property on="DB Camera Config" class="Bool (strict)"("Strings [4]"=w364) -> ()  [unwired: 2 in, 2 out]
      }
      event "Motor.Enable": Value Change {
        n226 = event-data() -> ("NewVal"=w372:bool)  [unwired: 1 in]
        n227 = Unbundle("Motor") -> ("Value"=w371:dbl)  [unwired: 1 out]
        n228 = Select(t=w371, s=w372, f=0.0) -> (s? t:f=w369:dbl)
        n229 = call <vilib>:"NT Write Number.vi"("Numeric"=w369, "Name"=w368) -> ()  [unwired: 9 in, 1 out]
      }
      event "Test Slider": Value Change {
        n230 = event-data() -> ("NewVal"=w375:dbl)  [unwired: 1 in]
        n231 = call <vilib>:"NT Write Number.vi"("Numeric"=w375, "Name"=w376) -> ()  [unwired: 9 in, 1 out]
      }
      event "On/Off": Value Change {
        n232 = event-data() -> ("NewVal"=w380:bool)  [unwired: 1 in]
        n233 = Boolean To (0,1)(Boolean=w380) -> (0, 1=w379:i16)
        n234 = call <vilib>:"NT Write Number.vi"("Numeric"=w379, "Name"=w378) -> ()  [unwired: 9 in, 1 out]
      }
      event "Rev/Fwd": Value Change {
        n235 = event-data() -> ("NewVal.Forward"=w388:bool, "NewVal.Reverse"=w387:bool)  [unwired: 1 in]
        n236 = Boolean To (0,1)(Boolean=w388) -> (0, 1=w384:i16)
        n237 = Boolean To (0,1)(Boolean=w387) -> (0, 1=w386:i16)
        n238 = Negate(x=w386) -> (-x=w385:i16)
        n239 = Add(x=w384, y=w385) -> (x+y=w383:i16)
        n240 = call <vilib>:"NT Write Number.vi"("Numeric"=w383, "Name"=w382) -> ()  [unwired: 9 in, 1 out]
      }
      event "Test Ring": Value Change {
        n241 = event-data() -> ("NewVal"=w392:u16)  [unwired: 1 in]
        n242 = property on="Test Ring" class="Ring (strict)"() -> ("Strings []"=w393:string[])  [unwired: 2 in, 2 out]
        n243 = Index Array(array=w393, index=w392) -> (element=w391:string)
        n244 = call <vilib>:"NT Write String.vi"("String"=w391, "Name"=w390) -> ()  [unwired: 9 in, 1 out]
      }
      event "Rec Mode": Value Change {
        # "Update globals for recording mode and path to read log from.\nClear when logging and let NetworkTables set path for vision to\nuse."
        n245 = event-data() -> ("NewVal"=w403:enum32{"Stop", "Record", "Playback"})  [unwired: 1 in]
        n246 = global write "WPI_DashboardLogging Global.vi" "Logging Filename"(path "") -> ()
        n247 = case shown="\"Stop\", \"Record\"" w403 {
          tunnel: w402 -> [_ w405 w413]
          tunnel: [_ _ w412] -> w399
          tunnel: [_ _ w411] -> _
          tunnel: w397 -> [_ _ w409]
          tunnel: cluster{i32, i32} {-250, 170} -> [_ _ w408]
          tunnel: [_ _ T16 {"Image Size"=TRUE, "Image Type"=TRUE, "Pixel Value"=TRUE, "ROI Information"=TRUE, "Zoom Factor"=FALSE} ("Image Information Shown:All Elements")] -> w395
          tunnel: [_ _ TRUE ("Zoom Factor")] -> w394
          frame Default {
          }
          frame "Stop", "Record" {
            # "Place Window too"
            n248 = invoke class="VI" method="FP.Close"(reference=w405) -> (reference out=w404:refnum<vi>)  [unwired: 2 in, 2 out]
            n249 = invoke class="VI" method="Abort VI"(reference=w404) -> ()  [unwired: 2 in, 3 out]
          }
          frame "Playback" {
            n250 = call "Open Playback Panel.vi"("Offset"=w408, "DB VI Ref"=w409, "Playback in"=w413) -> ("Playback out"=w410:refnum<vi>)  [unwired: 8 in]
            n251 = register-events(w410) -> (reference out=w412:refnum<event-registration>, error out=w411:errorcluster)  [unwired: 2 in]
          }
        }
        n252 = global write "WPI_DashboardLogging Global.vi" "Recording"(w403) -> ()
        n253 = property on="Camera Image" class="ImageControl"("Image Information Shown"=w395, "Image Information Visible"=w394) -> ()  [unwired: 2 in, 2 out]
        n254 = call <vilib>:"WPI_DashboardNT Log FieldName Cache.vi"("Operation"=enum16{"Lookup/Add", "Index", "Clear"}."Clear") -> ()  [unwired: 8 in, 3 out]
      }
      event Panel Close {
        w414 = enum32{"Stop", "Record", "Playback"}."Stop" ("Rec Mode")
        n255 = event-data() -> ()  [unwired: 1 in, 4 out]
        n256 = local write "Rec Mode"(w414) -> ()
        n257 = global write "WPI_DashboardLogging Global.vi" "Recording"(w414) -> ()
      }
      event Panel Close {
        # "Abort playback window and ourself"
        n258 = event-data() -> ()  [unwired: 1 in, 4 out]
        n259 = invoke class="VI" method="FP.Close"(reference=w419) -> (reference out=w418:refnum<vi>)  [unwired: 2 in, 2 out]
        n260 = invoke class="VI" method="Abort VI"(reference=w418) -> (error out=w417:errorcluster)  [unwired: 2 in, 2 out]
        n261 = invoke class="VI" method="Abort VI"(error in=w417) -> ()  [unwired: 2 in, 3 out]
      }
    }
  }
  n262 = property on="On/Off" class="Bool (strict)"("Visible"=w38) -> ()  [unwired: 2 in, 2 out]
  n263 = property on="Motor" class="Clust (strict)"("Visible"=w38) -> ()  [unwired: 2 in, 2 out]
  n264 = property on="Progress" class="Clust (strict)"("Visible"=w38) -> ()  [unwired: 2 in, 2 out]
  n265 = property on="Test Ring" class="Ring (strict)"("Visible"=w38) -> ()  [unwired: 2 in, 2 out]
  n266 = property on="Rev/Fwd" class="Clust (strict)"("Visible"=w38) -> ()  [unwired: 2 in, 2 out]
  n267 = property on="Camera Settings" class="Clust (strict)"("Visible"=w38) -> ()  [unwired: 2 in, 2 out]
  n268 = local write "DB Camera Config"(w38) -> ()
  n269 = global write "WPI_DashboardLogging Global.vi" "Recording"(w21) -> ()
  n270 = local write "Rec Mode"(w21) -> ()
  n271 = local write "Drawback Pistons Activated"(TRUE) -> ()
  n272 = case shown="False" "Manual Mechanism Override" {
    frame False {
      n273 = local read "Are Grabber Pistons Extended"() -> (w420:bool)
      n274 = local read "Is The Firing Pin Piston Extended"() -> (w422:bool)
      n275 = local read "Are Drawback Pistons Extended"() -> (w421:bool)
      n276 = local write "Grabber Pistons Extended"(w420) -> ()
      n277 = local write "Firing Pin Piston Extended"(w422) -> ()
      n278 = local write "Drawback Piston Extended"(w421) -> ()
    }
    frame True {
    }
  }
  n279 = local read "Is The Firing Pin Piston Extended"() -> (w10:bool)
  n280 = local read "Firing Pin Piston Extended"() -> (w9:bool)
  n281 = local read "Are Drawback Pistons Extended"() -> (w11:bool)
  n282 = local read "Drawback Piston Extended"() -> (w12:bool)
  n283 = local read "Are Grabber Pistons Extended"() -> (w7:bool)
  n284 = local read "Grabber Pistons Extended"() -> (w8:bool)
  n285 = Equal?(x=w10, y=w9) -> (x = y?=w5:bool)
  n286 = Equal?(x=w12, y=w11) -> (x = y?=w6:bool)
  n287 = Equal?(x=w8, y=w7) -> (x = y?=w4:bool)
  n288 = And(x=w6, y=w5) -> (x .and. y?=w3:bool)
  n289 = And(x=w3, y=w4) -> (x .and. y?=w2:bool)
  n290 = local write "Buttons Of Same Pistons In Same State"(w2) -> ()
